vi "HF2LI_Monitor.vi"() -> ()   [LabVIEW 2019]
uses:
  Cryotum_ami_old/CryoTUM_AMI/sub_vi-s/Monitors/Utility/HF2LI/HF2LI.ctl
  Global/Global Variables/Data_Display_global.vi
  Equipment/Zurich Instruments LabOne/Public/Configure/ziGetValueDemodSampleEx.vi
  Equipment/Zurich Instruments LabOne/Public/Configure/ziGetValueDouble.vi
  Equipment/Zurich Instruments LabOne/Zurich Instruments LabOne.lvlib
panel:
  in  "stop":bool
  out "HF2LI-Cluster":T1
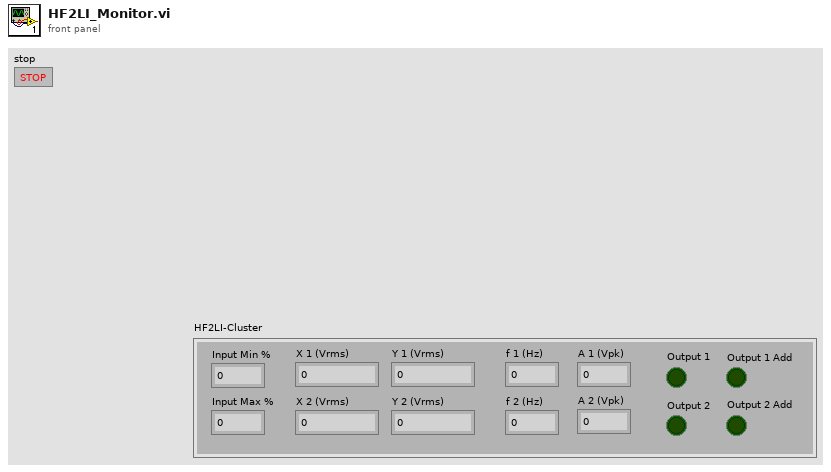
[diagram p1: front panel]
types:
  T1 = typedef "HF2LI.ctl" = cluster{"X 1 (Vrms)":dbl, "Y 1 (Vrms)":dbl, "A 1 (Vpk)":dbl, "A 2 (Vpk)":dbl, "Output 1":bool, "Output 2":bool, "f 1 (Hz)":dbl, "f 2 (Hz)":dbl, "X 2 (Vrms)":dbl, "Y 2 (Vrms)":dbl, "Output 1 Add":bool, "Output 2 Add":bool, "Input Min %":dbl, "Input Max %":dbl}
  T2 = cluster{"LIA7230-Running":bool, "LIA7230-Running 2":bool, "LIA7230-Running 3":bool, "SR830-Running":bool, "SR830-Running 2":bool, "SR830-Running 3":bool, "PE7265-running":bool, "zurich_Lock_in-running":bool, "HF2LI-Running":bool}
  T3 = typedef "Zurich Instruments LabOne.lvlib/ziTypeHandle.ctl" = cluster{"handleValid":bool, "Conn":u64, "Path Prefix":string, "Handle":u64, "Connected":bool, "Clockbase(s)":dbl}
  T4 = typedef "Zurich Instruments LabOne.lvlib/ziTypeDemodSampleSingle.ctl" = cluster{"Timestamps (ticks)":u64, "X (Vrms)":dbl, "Y (Vrms)":dbl, "Osc Phase (deg)":dbl, "Freq (Hz)":dbl, "DIO":u32, "AuxIn0 (V)":dbl, "AuxIn1 (V)":dbl, "Trigger":u32}
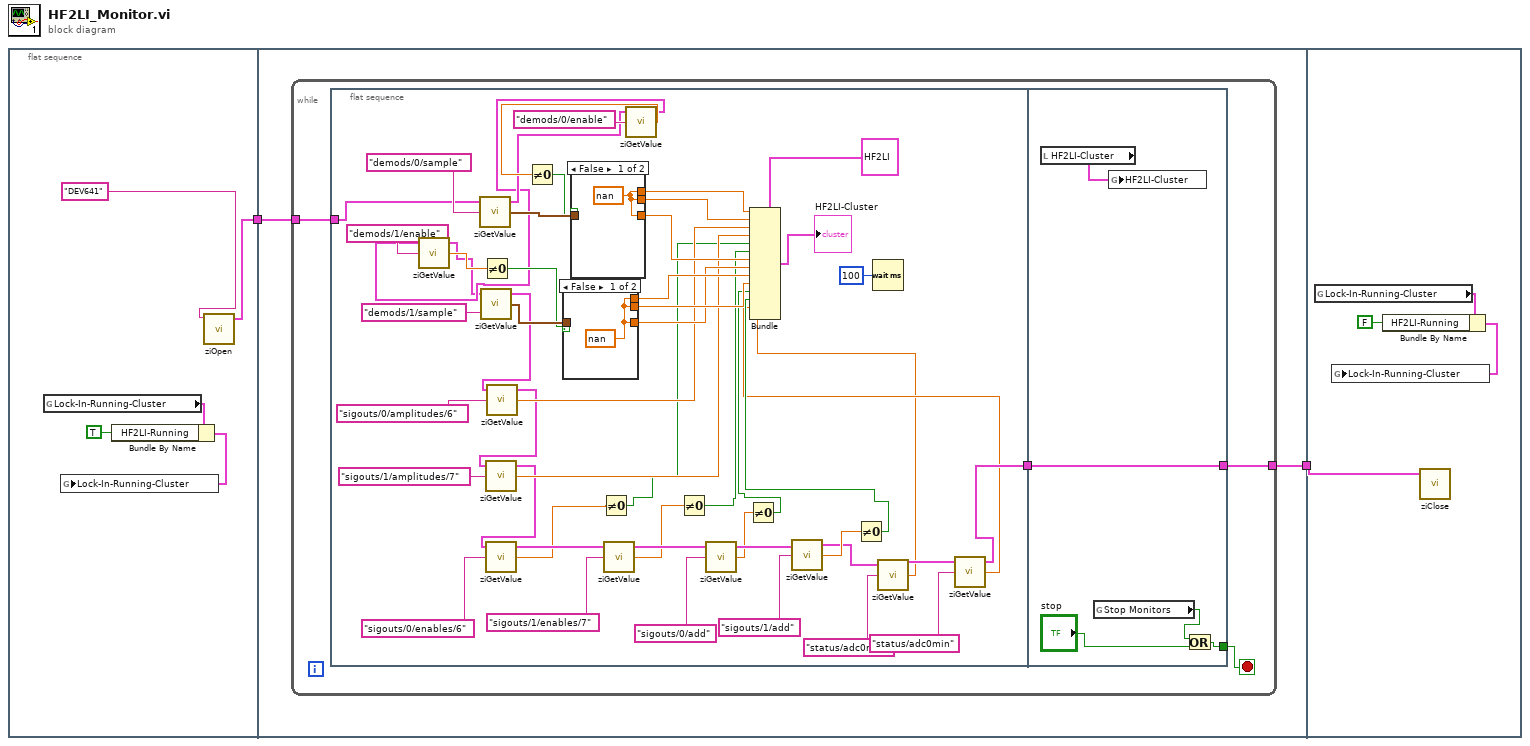
[diagram p0: block diagram]
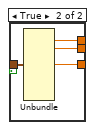
[diagram p2: hidden frame]
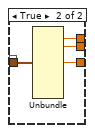
[diagram p3: hidden frame]
diagram:
  n1 = flat-sequence {
    tunnel: [w7] -> w2
    tunnel: w2 -> [w9]
    tunnel: [w8] -> w1
    tunnel: w1 -> [w84]
    frame #0 {
      n2 = global read "Data_Display_global.vi" "Lock-In-Running-Cluster"() -> (w3:T2)
      n3 = Bundle By Name(cluster=w3, "HF2LI-Running"=TRUE) -> (w4:T2)
      n4 = global write "Data_Display_global.vi" "Lock-In-Running-Cluster"(w4) -> ()
      n5 = call "ziOpen.vi"("Address"="DEV641") -> ("HandleOut"=w7:T3)  [unwired: 3 in, 2 out]
    }
    frame #1 {
      n6 = while {
        tunnel: w9 -> [w12]
        tunnel: [w11] -> w8
        stop <- w13 stop-if-true
        n7 = flat-sequence {
          tunnel: w12 -> [w52]
          tunnel: [w27] -> w10
          tunnel: [w80] -> w11
          tunnel: [w77] -> w13
          tunnel: w10 -> [w80]
          frame #0 {
            n8 = call-poly "ziGetValue.vi"("Path"="demods/0/sample", "Handle In"=w52) -> ("Demod Sample Out"=w61:T4, "Handle Out"=w16:T3)  [unwired: 1 in, 1 out]
            n9 = call-poly "ziGetValue.vi"("Path"="demods/0/enable", "Handle in"=w16) -> ("Value"=w19:dbl, "Handle out"=w15:T3)  [unwired: 1 in, 1 out]
            n10 = call-poly "ziGetValue.vi"("Path"="demods/1/enable", "Handle in"=w15) -> ("Value"=w18:dbl, "Handle out"=w14:T3)  [unwired: 1 in, 1 out]
            n11 = call-poly "ziGetValue.vi"("Path"="demods/1/sample", "Handle In"=w14) -> ("Demod Sample Out"=w62:T4, "Handle Out"=w49:T3)  [unwired: 1 in, 1 out]
            n12 = Not Equal To 0?(x=w18) -> (x != 0?=w17:bool)
            n13 = call-poly "ziGetValue.vi"("Path"="sigouts/0/amplitudes/6", "Handle in"=w49) -> ("Value"=w53:dbl, "Handle out"=w48:T3)  [unwired: 1 in, 1 out]
            n14 = call-poly "ziGetValue.vi"("Path"="sigouts/1/amplitudes/7", "Handle in"=w48) -> ("Value"=w50:dbl, "Handle out"=w43:T3)  [unwired: 1 in, 1 out]
            n15 = call-poly "ziGetValue.vi"("Path"="sigouts/0/enables/6", "Handle in"=w43) -> ("Value"=w37:dbl, "Handle out"=w42:T3)  [unwired: 1 in, 1 out]
            n16 = Not Equal To 0?(x=w19) -> (x != 0?=w20:bool)
            n17 = case shown="False" w17 {
              tunnel: w62 -> [_ w70]
              tunnel: [w66 w69] -> w58
              tunnel: [w66 w68] -> w57
              tunnel: [w66 w67] -> w56
              frame False {
                w66 = nan
              }
              frame True {
                n18 = Unbundle(w70) -> ("X (Vrms)"=w69:dbl, "Y (Vrms)"=w68:dbl, "Freq (Hz)"=w67:dbl)  [unwired: 6 out]
              }
            }
            n19 = case shown="False" w20 {
              tunnel: w61 -> [_ w75]
              tunnel: [w71 w74] -> w60
              tunnel: [w71 w73] -> w59
              tunnel: [w71 w72] -> w55
              frame False {
                w71 = nan
              }
              frame True {
                n20 = Unbundle(w75) -> ("X (Vrms)"=w74:dbl, "Y (Vrms)"=w73:dbl, "Freq (Hz)"=w72:dbl)  [unwired: 6 out]
              }
            }
            n21 = Not Equal To 0?(x=w37) -> (x != 0?=w36:bool)
            n22 = call-poly "ziGetValue.vi"("Path"="sigouts/1/enables/7", "Handle in"=w42) -> ("Value"=w35:dbl, "Handle out"=w41:T3)  [unwired: 1 in, 1 out]
            n23 = Not Equal To 0?(x=w35) -> (x != 0?=w34:bool)
            n24 = call-poly "ziGetValue.vi"("Path"="sigouts/0/add", "Handle in"=w41) -> ("Value"=w33:dbl, "Handle out"=w40:T3)  [unwired: 1 in, 1 out]
            n25 = Not Equal To 0?(x=w33) -> (x != 0?=w32:bool)
            n26 = call-poly "ziGetValue.vi"("Path"="sigouts/1/add", "Handle in"=w40) -> ("Value"=w31:dbl, "Handle out"=w29:T3)  [unwired: 1 in, 1 out]
            n27 = Not Equal To 0?(x=w31) -> (x != 0?=w30:bool)
            n28 = Wait (ms)(milliseconds to wait=u32 100) -> ()  [unwired: 1 out]
            n29 = call-poly "ziGetValue.vi"("Path"="status/adc0max", "Handle in"=w29) -> ("Value"=w23:dbl, "Handle out"=w28:T3)  [unwired: 1 in, 1 out]
            n30 = call-poly "ziGetValue.vi"("Path"="status/adc0min", "Handle in"=w28) -> ("Value"=w24:dbl, "Handle out"=w27:T3)  [unwired: 1 in, 1 out]
            n31 = Bundle(cluster=T1 {"X 1 (Vrms)"=2.7056741238785867e-06, "Y 1 (Vrms)"=-1.312399113553479e-06, "A 1 (Vpk)"=0.39999694821890425, "A 2 (Vpk)"=0.04999580380099335, "Output 1"=FALSE, "Output 2"=FALSE, "f 1 (Hz)"=201.99999966052928, "f 2 (Hz)"=201.99999966052928, "X 2 (Vrms)"=3.017847906110667e-06, "Y 2 (Vrms)"=-2.261753825762805e-06, "Output 1 Add"=FALSE, "Output 2 Add"=FALSE, "Input Min %"=0.0, "Input Max %"=0.0} ("HF2LI-Cluster"), "X 1 (Vrms)"=w60, "Y 1 (Vrms)"=w59, "A 1 (Vpk)"=w53, "A 2 (Vpk)"=w50, "Output 1"=w36, "Output 2"=w34, "f 1 (Hz)"=w55, "f 2 (Hz)"=w56, "X 2 (Vrms)"=w58, "Y 2 (Vrms)"=w57, "Output 1 Add"=w32, "Output 2 Add"=w30, "Input Min %"=w24, "Input Max %"=w23) -> (→"HF2LI-Cluster":T1)
          }
          frame #1 {
            n32 = local read "HF2LI-Cluster"() -> (w76:T1)
            n33 = global read "Data_Display_global.vi" "Stop Monitors"() -> (w79:bool)
            n34 = global write "Data_Display_global.vi" "HF2LI-Cluster"(w76) -> ()
            n35 = Or(x=w79, y="stop") -> (x .or. y?=w77:bool)
          }
        }
      }
    }
    frame #2 {
      n36 = global read "Data_Display_global.vi" "Lock-In-Running-Cluster"() -> (w81:T2)
      n37 = Bundle By Name(cluster=w81, "HF2LI-Running"=FALSE) -> (w82:T2)
      n38 = global write "Data_Display_global.vi" "Lock-In-Running-Cluster"(w82) -> ()
      n39 = call "ziClose.vi"("Handle In"=w84) -> ()  [unwired: 3 in, 2 out]
    }
  }
